vi "ITSERP-Application-Dir-Support.vi"(0 "Support Resource Relative Filepath":string, 11 "error in":errorcluster) -> (4 "Support Filepath":path, 6 "appended path 2":path, 15 "error out":errorcluster)   [LabVIEW 2013]
uses:
  ERP-Container/ERP-ConfigPageNewFeather/PCert-ConfigPageNF.lvclass
panel:
  out "Deploy Root":path
  out "Provider Root":path
  out "appended path":path
  # "Inputs"
  # "Outputs"
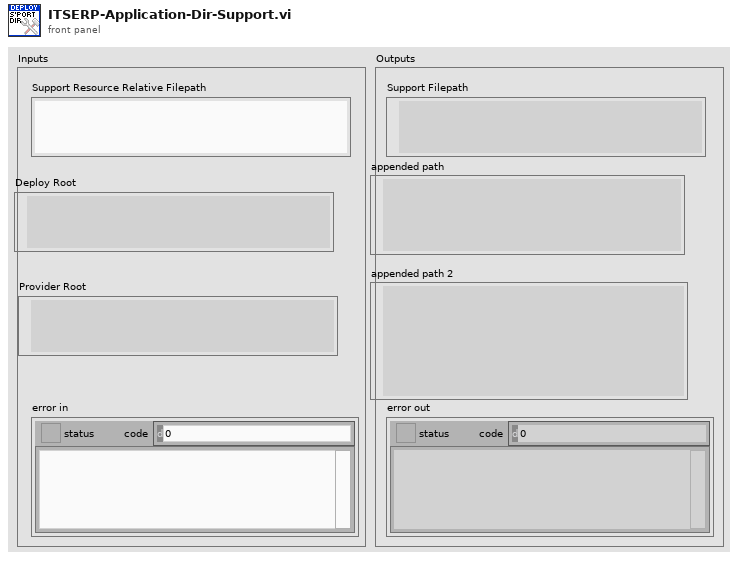
[diagram p1: front panel]
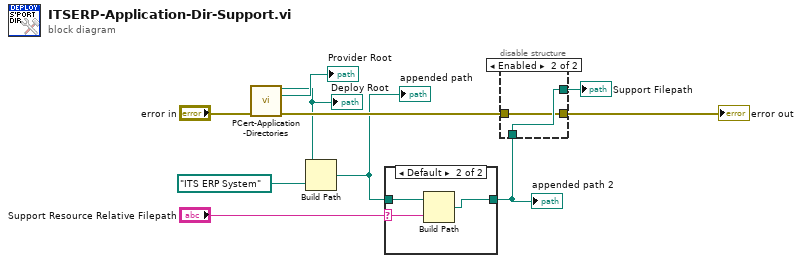
[diagram p0: block diagram]
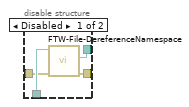
[diagram p2: hidden frame]
diagram:
  n1 = call "PCert-Application-Directories.vi"("error in"="error in") -> ("Deploy Root"=w2:path, "Provider Root"=→"Provider Root":path, "error out"=w5:errorcluster)  [unwired: 12 in]
  "Deploy Root" <- w2
  n2 = Build Path(base path=w2, name or relative path=path "ITS ERP System") -> (appended path=w1:path)
  "appended path" <- w1
  n3 = case shown="Default" "Support Resource Relative Filepath" {
    selector: "Support Resource Relative Filepath" -> [_ w12]
    tunnel: [w11 w14] -> w7
    tunnel: w1 -> [w11 w13]
    frame "" {
    }
    frame Default {
      n4 = Build Path(base path=w13, name or relative path=w12) -> (appended path=w14:path)
    }
  }
  "appended path 2" <- w7
  n5 = disable-structure shown="Enabled" {
    disable-tunnel: w7 -> [w18 w20]
    disable-tunnel: [w17 w20] -> w6
    disable-tunnel: w5 -> [w16 w19]
    disable-tunnel: [w15 w19] -> w4
    frame Disabled {
      n6 = call "FTW-File-DereferenceNamespace.vi"("error in"=w16, "Base Filepath"=w18) -> ("error out"=w15:errorcluster, "Actual Filepath"=w17:path)  [unwired: 8 in]
    }
    frame Enabled {
    }
  }
  "error out" <- w4
  "Support Filepath" <- w6
